vi "WinCI Get Provider DLL Path.vi"(8 "error in (no error)":errorcluster, 10 "SCC provider key":string) -> (0 "error out":errorcluster, 2 "provider dll path":string, 3 "provider name":string)   [LabVIEW 2017, in "NI_SCC_WinCI.lvlib"]
uses:
  <vilib>/SourceControl/Providers/WinCI/NI_SCC_WinCI.lvlib
  <vilib>/registry/registry.llb/Registry SAM.ctl
  <vilib>/registry/registry.llb/Read Registry Value Simple STR.vi
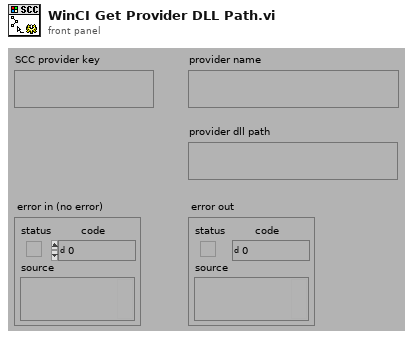
[diagram p1: front panel]
types:
  T1 = typedef "Registry SAM.ctl" = enum32{"KEY_QUERY_VALUE", "KEY_SET_VALUE", "KEY_CREATE_SUB_KEY", "KEY_ENUMERATE_SUB_KEYS", "KEY_NOTIFY", "KEY_CREATE_LINK", "KEY_READ", "KEY_WRITE", "KEY_ALL_ACCESS", "KEY_READ | KEY_WRITE"}
  T2 = typedef "Registry refnum.ctl" = refnum<k1>
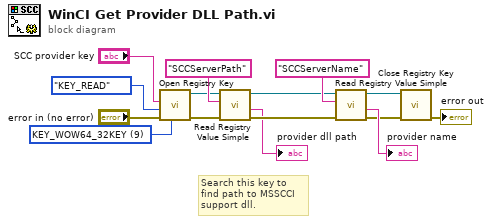
[diagram p0: block diagram]
diagram:
  w1 = u16 9 items=["DEFAULT"=0, "KEY_WOW64_64KEY"=8, "KEY_WOW64_32KEY"=9] ("alternate registry view mask")
  # "Search this key to find path to MSSCCI support dll."
  n1 = call <vilib>:"Open Registry Key.vi"("registry view"=w1, "error in (no error)"="error in (no error)", "security access mask (KEY_READ | KEY_WRITE)"=Registry_SAM."KEY_READ", "subkey"="SCC provider key") -> ("error out"=w7:errorcluster, "refnum out"=w6:T2)  [unwired: 1 in, 5 out]
  n2 = call-poly <vilib>:"Read Registry Value Simple.vi"("error in (no error)"=w7, "value"="SCCServerPath", "refnum"=w6) -> ("error out"=w11:errorcluster, "String/Binary data"=→"provider dll path":string, "refnum out"=w10:T2)  [unwired: 1 in, 3 out]
  n3 = call-poly <vilib>:"Read Registry Value Simple.vi"("error in (no error)"=w11, "value"="SCCServerName", "refnum"=w10) -> ("error out"=w13:errorcluster, "String/Binary data"=→"provider name":string, "refnum out"=w12:T2)  [unwired: 1 in, 3 out]
  n4 = call <vilib>:"Close Registry Key.vi"("error in (no error)"=w13, "refnum"=w12) -> ("error out"=→"error out":errorcluster)  [unwired: 5 out]
